vi "DN4_Counter_RegisterLVEvent.vi"(3 "error in (no error)":errorcluster, 4 "CntrEvent":refnum<user-event>, 5 "Task ID":u32) -> (0 "error out":errorcluster, 1 "CntrEvent":refnum<user-event>, 2 "Task ID":u32)   [LabVIEW 2009]
uses:
  Windows/System32/AdvLvDaq.dll
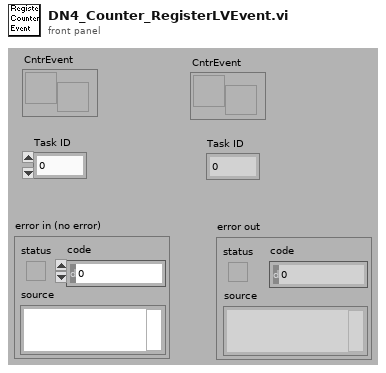
[diagram p1: front panel]
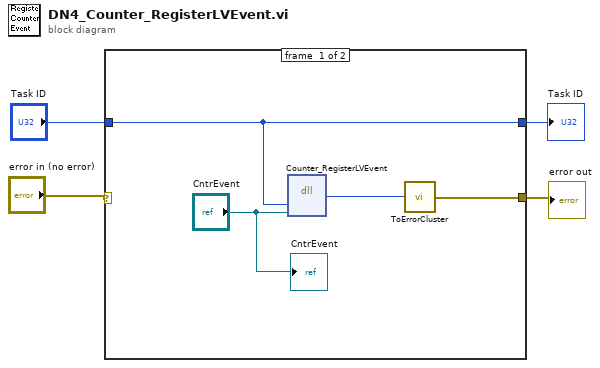
[diagram p0: block diagram]
diagram:
  n1 = case shown="No Error" "error in (no error)" {
    selector: "error in (no error)" -> [_ w10]
    tunnel: [w6 w10] -> w3
    tunnel: "Task ID" -> [w5 w9]
    tunnel: [w5 w9] -> w1
    frame #0 {
      n2 = dll-call lib="C:/Windows/System32/AdvLvDaq.dll" fn="Counter_RegisterLVEvent"("taskId"=w5, "cntrEvent"="CntrEvent") -> ("return type"=w7:i32)  [unwired: 4 in, 3 out]
      n3 = call <userlib>:"ToErrorCluster.vi"("error code"=w7) -> ("error out"=w6:errorcluster)
      "CntrEvent" <- "CntrEvent"
    }
    frame #1 {
    }
  }
  "error out" <- w3
  "Task ID" <- w1
